vi "ReadConfigFile.vi"(0 "reference in":refnum<class "DAQ_Base.lvclass">, 1 "ConfigFlieName":string="DAQSetting.ini", 5 "error in (no error)":errorcluster) -> (14 "reference out":refnum<class "DAQ_Base.lvclass">, 19 "error out":errorcluster)   [LabVIEW 2020, in "DAQ.lvlib" / "DAQ_Base.lvclass"]
uses:
  DAQ_Base.lvclass
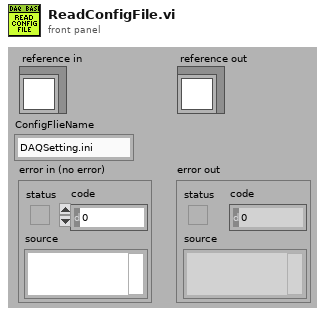
[diagram p1: front panel]
types:
  T1 = typedef "DAQ.lvlib/DAQ_Base.lvclass/ObjectAttributesRef.ctl" = refnum<data-value>
  T2 = typedef "DAQ.lvlib/DAQ_Base.lvclass/ObjectAttributes.ctl" = cluster{"MyAttribute":dbl, "RootPath":path, "DAQSettings":T3, "DaqCollector":cluster{"CollectDataQueue":refnum<queue>, "ArryDataCollectorChannel":T9[], "RealTimeValues":dbl[]}, "CollectorChannelEnable":bool[]}
  T3 = typedef "DAQ.lvlib/DAQ_Base.lvclass/DAQSettings.ctl" = cluster{"SampleSettings":T4, "AI_ChannelSettings":T5, "AO_ChannelSettings":T7, "Cnt_ChannelSettings":T8}
  T4 = typedef "DAQ.lvlib/DAQ_Base.lvclass/SampleSettings.ctl" = cluster{"samples per channel":i32, "SampleRate":dbl, "TansMaxLength":dbl, "ReadTimeOut":dbl, "时钟源":tag}
  T5 = typedef "DAQ.lvlib/DAQ_Base.lvclass/AI_ChannelSettings.ctl" = cluster{"AI_SettingsArry":cluster{"DeviceName":tag, "physical channels":tag, "AssignName":string, "输入信号类型":T6, "Max_value":dbl, "Min_value":dbl, "单位":i32, "shunt resistor location":i32, "external shunt resistor value":dbl, "标定系数":cluster{"Scale":dbl, "Offset":dbl}}[]}
  T6 = typedef "AI信号类型.ctl" = i32
  T7 = typedef "DAQ.lvlib/DAQ_Base.lvclass/AO_ChannelSettings.ctl" = cluster{"布尔":bool}
  T8 = typedef "DAQ.lvlib/DAQ_Base.lvclass/Cnt_ChannelSettings.ctl" = cluster{"Cnt_ChannelSettings":cluster{"类型":enum16{"Linear", "Rotate"}, "CounterNbr":tag, "AssignName":string, "单位":u16, "decoding type":u16, "PPR_DistancePerPulse":dbl, "Initial Position ":dbl, "z index enable":bool, "z index phase":i32, "source":tag}[]}
  T9 = typedef "DAQ.lvlib/DAQ_Base.lvclass/DataCollector.ctl" = cluster{"DataCollectArry":dbl[][], "Update":bool}
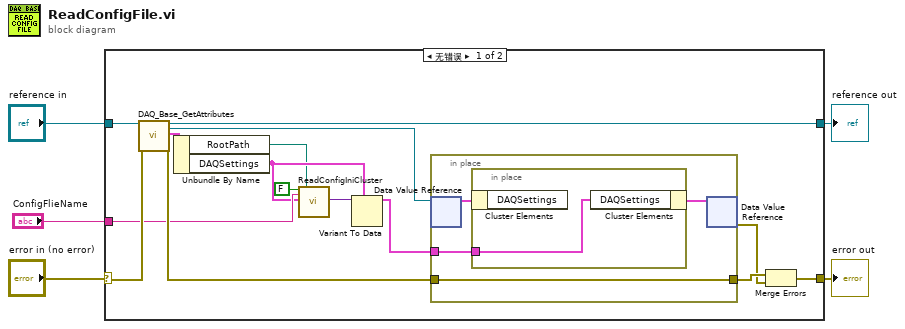
[diagram p0: block diagram]
diagram:
  n1 = case shown="无错误" "error in (no error)" {
    selector: "error in (no error)" -> [w17 w27]
    tunnel: [w20 w27] -> w4
    tunnel: [w18 w26] -> w2
    tunnel: "reference in" -> [w19 w26]
    tunnel: "ConfigFlieName" -> [w10 _]
    frame No Error {
      n2 = call "DAQ_Base_GetAttributes.vi"("reference in"=w19, "error in (no error)"=w17) -> ("reference out"=w18:refnum<class "DAQ_Base.lvclass">, "attributes ref"=w12:T1, "attributes"=w15:T2, "error out"=w16:errorcluster)  [unwired: 14 in]
      n3 = Unbundle By Name(w15) -> ("RootPath"=w6:path, "DAQSettings"=w8:T3)
      n4 = call "ReadConfigIniCluster.vi"("更随产品型号变更？"=FALSE, "ConfigFlieName"=w10, "ConfigOut"=w8, "根路径"=w6) -> ("ConfigOut"=w9:variant)  [unwired: 14 in, 1 out]
      n5 = Variant To Data(type=w8, Variant=w9) -> (data=w7:T3)  [unwired: 1 in, 1 out]
      n6 = in-place {
        in-place-border: w16 -> [w22]
        in-place-border: [w22] -> w14
        in-place-border: w7 -> [w21]
        n7 = in-place-dvr #1(w12) -> (w23:T2)  [unwired: 1 out]
        n8 = in-place {
          in-place-border: w21 -> [w25]
          n9 = in-place-cluster #2(w23) -> ()  [unwired: 1 out]
          n10 = in-place-cluster #2("DAQSettings"=w25) -> (w24:T2)
        }
        n11 = in-place-dvr #1(w24) -> (w13:errorcluster)  [unwired: 1 out]
      }
      n12 = Merge Errors(w14, w13) -> (w20:errorcluster)
    }
    frame Error {
    }
  }
  "error out" <- w4
  "reference out" <- w2
